vi "ExternalFOV.vi"(11 "Refnum in":T1) -> ()   [LabVIEW 2011]
uses:
  <vilib>/vision/Image Controls.llb/IMAQ Image.ctl
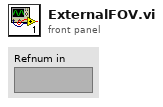
[diagram p1: front panel]
types:
  T1 = typedef "IMAQ Image.ctl" = refnum<image>
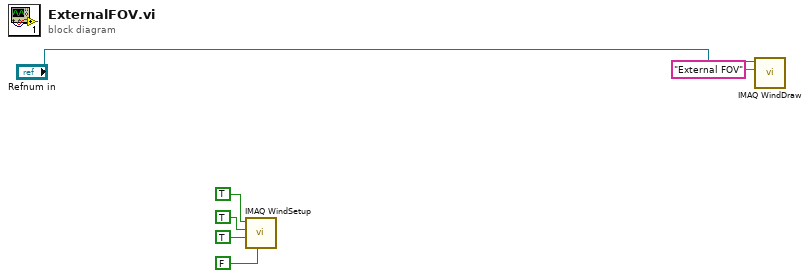
[diagram p0: block diagram]
diagram:
  n1 = call "IMAQ WindSetup"("Window is floating? (No)"=FALSE, "Window has title bar? (Yes)"=TRUE, "Window can close? (Yes)"=TRUE, "Window can grow? (Yes)"=TRUE) -> ()  [unwired: 7 in, 1 out]
  n2 = call "IMAQ WindDraw"("Title"="External FOV", "Image"="Refnum in") -> ()  [unwired: 8 in, 2 out]
